vi "opencvSegmentConvertCoordinatesAddZ.vi"(1 "XY":u16[][][](array[numeric])) -> (0 "XYZ":i32[][](array[numeric]))   [LabVIEW 2017]
panel:
  # "XY[frame,neuron,coordinate]"
  # "XYZ[neuron,coordinate]"
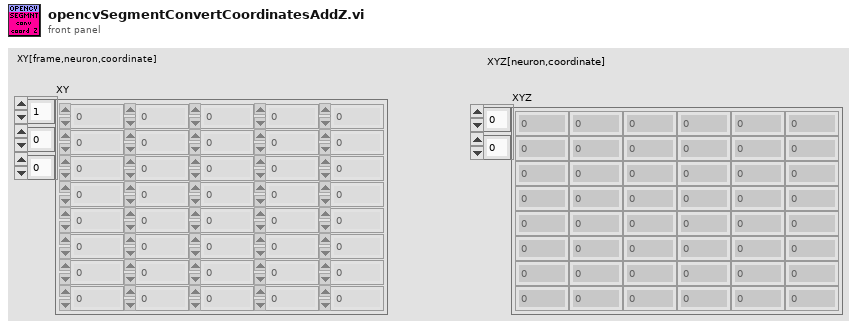
[diagram p1: front panel]
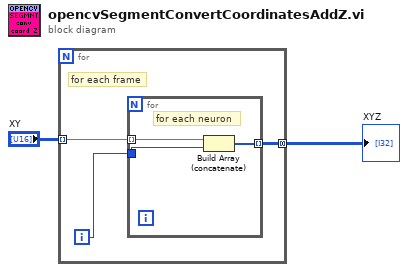
[diagram p0: block diagram]
diagram:
  n1 = for {
    tunnel: "XY" -> [w5] mode=indexing
    tunnel: [w4] -> w1 mode=concatenating
    i -> [w3]
    # "for each frame"
    n2 = for {
      tunnel: w5 -> [w8] mode=indexing
      tunnel: [w6] -> w4 mode=indexing
      tunnel: w3 -> [w7]
      # "for each neuron"
      n3 = Build Array (concatenate)(w8, w7) -> (w6:i32[])
    }
  }
  "XYZ" <- w1
